vi "TW Edit - Stage 1.vi"(6 "Text color":u32(colorbox), 7 "Icon Text":string, 8 "error in":errorcluster, 9 "Background":u32(colorbox)=7208704, 10 "New Subname":string, 11 "Template Project Path":path) -> (0 "error out":errorcluster, 4 "Result for debugging":cluster{"Name":string, picture[]}[](array[cluster]))   [LabVIEW 2021, in "Plugin Generator.lvlib"]
uses:
  Plugin Generator.lvlib
  <vilib>/CIF Foundation/CIF LabVIEW Scripting/LV Scripting/LV Scripting Utilities.lvlib
panel:
  in  "Debug":bool
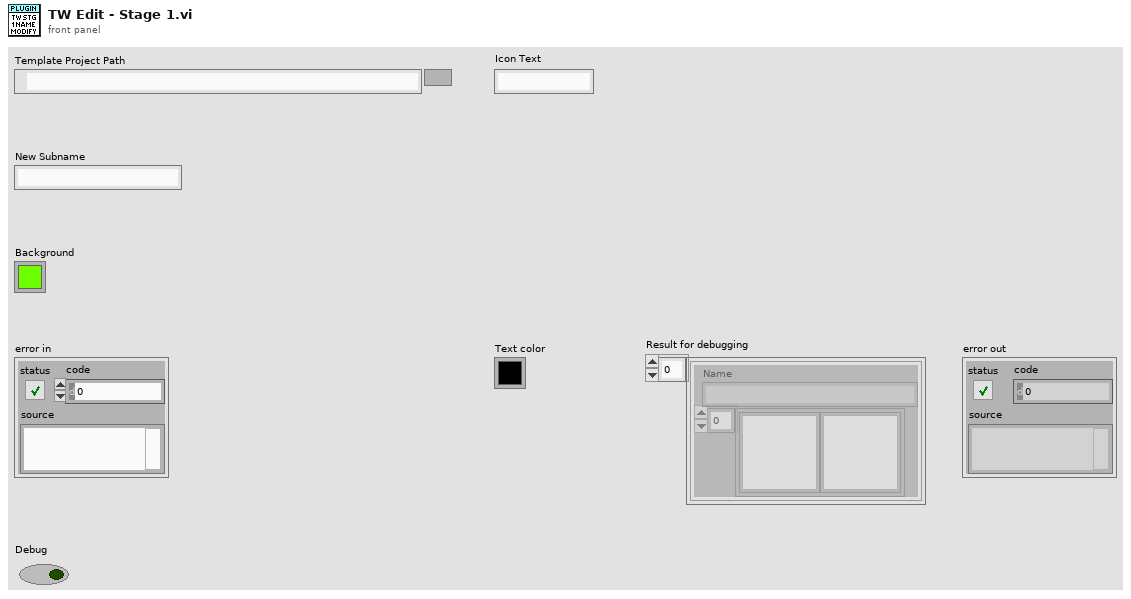
[diagram p1: front panel]
types:
  T1 = cluster{"Library Name":string, "Update Folder Name":bool}[]
  T2 = typedef "LV Scripting Utilities.lvlib/Target References.ctl" = cluster{"Target Reference":refnum<vi>, "VI References":refnum<vi>[], "Library References":refnum<vi>[], "Build References":refnum<vi>[]}
  T3 = typedef "LV Scripting Utilities.lvlib/Library Map.ctl" = map{string, refnum<vi>}
  T4 = typedef "LV Scripting Utilities.lvlib/VI Map.ctl" = map{string, refnum<vi>}
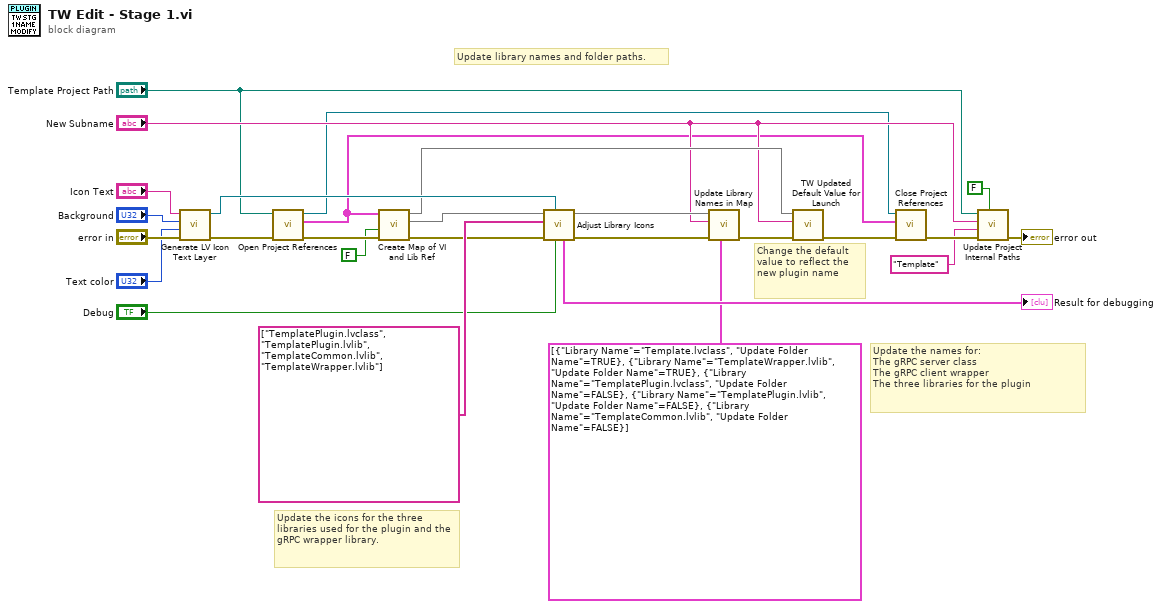
[diagram p0: block diagram]
diagram:
  # "Update library names and folder paths."
  # "Change the default value to reflect the new plugin name"
  # "Update the names for:\nThe gRPC server class\nThe gRPC client wrapper\nThe three libraries for the plugin"
  # "Update the icons for the three libraries used for the plugin and the gRPC wrapper library."
  n1 = call <vilib>:"Generate LV Icon Text Layer.vi"("error in (no error)"="error in", "Text color"="Text color", "Background"="Background", "Name"="Icon Text") -> ("error out"=w8:errorcluster, "Icon.lvlclass out"=w20:refnum<class "Icon.lvclass">)  [unwired: 5 in, 1 out]
  n2 = call <vilib>:"Open Project References.vi"("error in"=w8, "Project Path"="Template Project Path") -> ("error out"=w7:errorcluster, "VI, Library, and Build References"=w4:T2[], "Project Reference"=w5:refnum<vi>)  [unwired: 7 in]
  n3 = call <vilib>:"Create Map of VI and Lib Ref.vi"("error in"=w7, "RT Target"=FALSE, "VI, Library, and Build References"=w4) -> ("error out"=w19:errorcluster, "Library Map"=w21:T3, "VI Map"=w13:T4)  [unwired: 5 in, 1 out]
  n4 = call <vilib>:"Adjust Library Icons.vi"("Debug"="Debug", "Overlay Icon"=w20, "error in"=w19, "Library Names"=string[] ["TemplatePlugin.lvclass", "TemplatePlugin.lvlib", "TemplateCommon.lvlib", "TemplateWrapper.lvlib"], "Library Map in"=w21) -> ("error out"=w16:errorcluster, "Library Map out"=w17:map{string, refnum<vi>}, "Result for debugging"=→"Result for debugging":cluster{"Name":string, picture[]}[])  [unwired: 4 in]
  n5 = call <vilib>:"Update Library Names in Map.vi"("Libraries"=T1 [{"Library Name"="Template.lvclass", "Update Folder Name"=TRUE}, {"Library Name"="TemplateWrapper.lvlib", "Update Folder Name"=TRUE}, {"Library Name"="TemplatePlugin.lvclass", "Update Folder Name"=FALSE}, {"Library Name"="TemplatePlugin.lvlib", "Update Folder Name"=FALSE}, {"Library Name"="TemplateCommon.lvlib", "Update Folder Name"=FALSE}], "error in"=w16, "New Subname"="New Subname", "Library Map"=w17) -> ("error out"=w14:errorcluster)  [unwired: 6 in, 1 out]
  n6 = call "TW Updated Default Value for Launch.vi"("error in"=w14, "New Subname"="New Subname", "Name to VI Map"=w13) -> ("error out"=w6:errorcluster)  [unwired: 8 in]
  n7 = call <vilib>:"Close Project References.vi"("error in"=w6, "VI, Library, and Build References"=w4, "Project Reference"=w5) -> ("error out"=w3:errorcluster)  [unwired: 8 in]
  n8 = call <vilib>:"Update Project Internal Paths.vi"("Rename Project"=FALSE, "error in (no error)"=w3, "Replace Subname"="Template", "New Subname"="New Subname", "Project Path"="Template Project Path") -> ("error out"=→"error out":errorcluster)  [unwired: 6 in]
